vi "Cecília Questão 5.vi"() -> ()   [LabVIEW 2019]
uses:
  <vilib>/Analysis/5stat.llb/RMS (DBL).vi
  <vilib>/Utility/file.llb/Read Delimited Spreadsheet (DBL).vi
  <vilib>/Analysis/NI_AALPro.lvlib
panel:
  in  "Rodar VI":bool
  in  "Arquivo .txt":path=path "C:/Users/fmce520/Desktop/waveform.txt"
  out "SINAL COMPLETO":dbl[](graph)
  in  "Início dos valores numéricos \n(caracteres aparecem no gráfico com o valor 0)":i32=53
  in  "Threshold":dbl
  out "PULSO CAPTADO":cluster{i32[], dbl[]}(graph)
  out "Valor rms":dbl format="%0.2f"
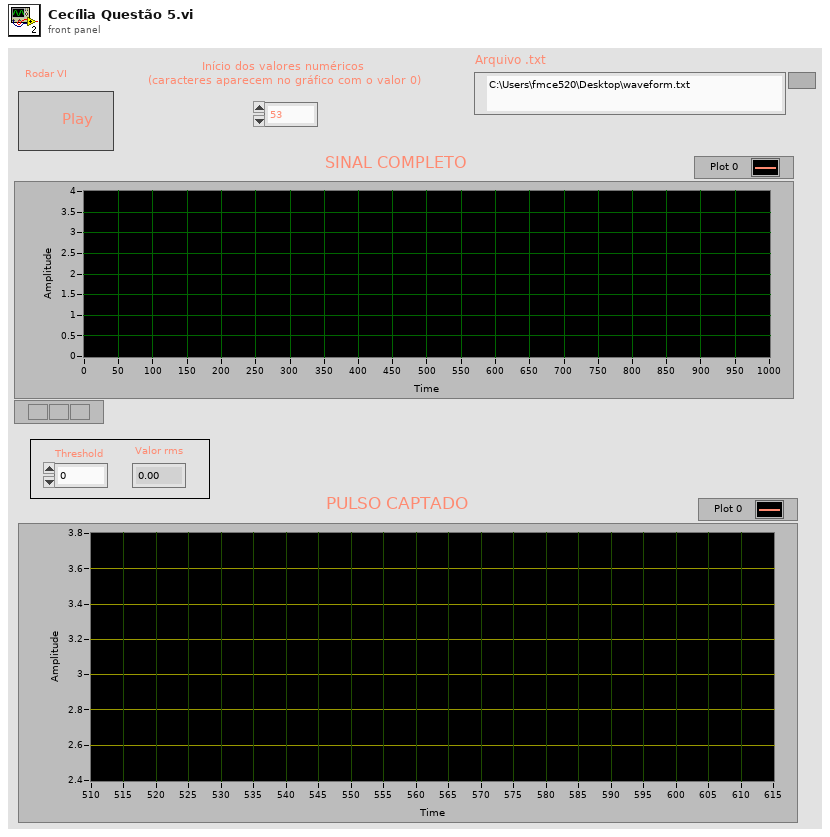
[diagram p1: front panel]
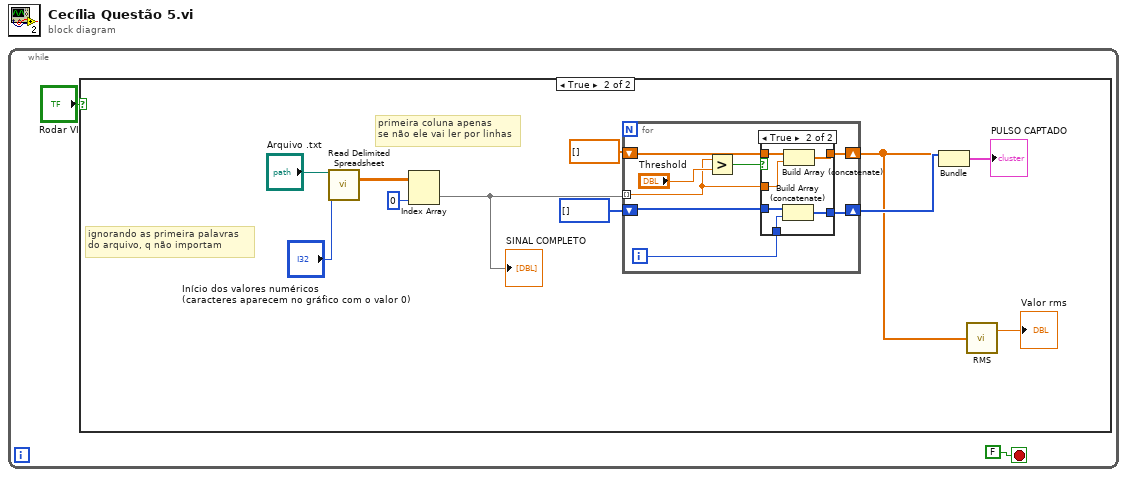
[diagram p0: block diagram]
diagram:
  n1 = while {
    stop <- FALSE stop-if-true
    n2 = case shown="True" "Rodar VI" {
      frame False {
      }
      frame True {
        # "ignorando as primeira palavras \ndo arquivo, q não importam"
        # "primeira coluna apenas\nse não ele vai ler por linhas"
        n3 = call-poly <vilib>:"Read Delimited Spreadsheet.vi"("file path (dialog if empty)"="Arquivo .txt", "start of read offset (chars.:0)"="Início dos valores numéricos \n(caracteres aparecem no gráfico com o valor 0)") -> ("all rows"=w12:dbl[][])  [unwired: 8 in, 5 out]
        n4 = Index Array(array=w12, index (col)=0 ("disabled index (col)")) -> (element=w5:dbl[])  [unwired: 1 in]
        "SINAL COMPLETO" <- w5
        n5 = for {
          tunnel: w5 -> [w18] mode=indexing
          shift-right: [w20] -> w3
          shift-left: dbl[] [] -> [w21]
          shift-right: [w16] -> w7
          shift-left: i32[] [] -> [w14]
          i -> [w15]
          n6 = Greater?(x=w18, y="Threshold") -> (0:w17:bool)
          n7 = case shown="True" w17 {
            tunnel: w21 -> [w23 w29]
            tunnel: [w23 w28] -> w20
            tunnel: w18 -> [_ w27]
            tunnel: [w22 w26] -> w16
            tunnel: w15 -> [_ w25]
            tunnel: w14 -> [w22 w24]
            frame False {
            }
            frame True {
              n8 = Build Array (concatenate)(w24, w25) -> (w26:i32[])
              n9 = Build Array (concatenate)(w29, w27) -> (w28:dbl[])
            }
          }
        }
        n10 = Bundle(w7, w3) -> (→"PULSO CAPTADO":cluster{i32[], dbl[]})  [unwired: 1 in]
        n11 = call-poly <vilib>:"RMS.vi"("X"=w3) -> ("rms value"=→"Valor rms":dbl)  [unwired: 1 out]
      }
    }
  }
